vi "Generate write queue item.vi"(8 "error in (no error)":errorcluster, 11 "Abort JSON in":refnum<class "Abort JSON.lvclass">) -> (0 "error out":errorcluster, 2 "Write queue item":T1, 3 "Abort JSON out":refnum<class "Abort JSON.lvclass">)   [LabVIEW 2020, in "wamplv.lvlib" / "Abort JSON.lvclass"]
uses:
  Abort JSON.lvclass
  Abort JSON.lvclass/Abort JSON.ctl
  f2b6dabe-d674-4de4-8983-0b42131ca8da.vi
  cf9281e4-cdc7-4391-bfc3-c4a2100e25ce.vi
  TypeDefs/Transport type.ctl
  wamplv.lvlib
  WAMP Client/Private/TypeDef/Write queue item.ctl
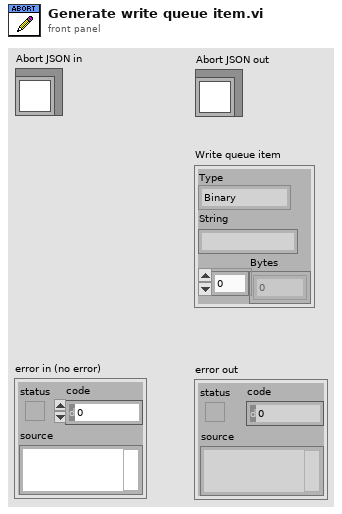
[diagram p1: front panel]
types:
  T1 = typedef "wamplv.lvlib/Write queue item.ctl" = cluster{"Type":T2, "String":string, "Bytes":u8[]}
  T2 = typedef "wamplv.lvlib/Transport type.ctl" = enum16{"Binary", "Text"}
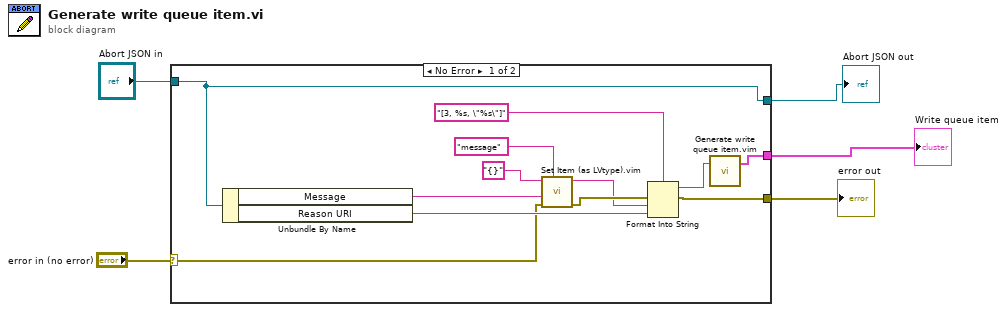
[diagram p0: block diagram]
diagram:
  n1 = case shown="No Error" "error in (no error)" {
    selector: "error in (no error)" -> [w10 w19]
    tunnel: "Abort JSON in" -> [w8 w18]
    tunnel: [w9 w19] -> w3
    tunnel: [w8 w18] -> w2
    tunnel: [w6 _] -> w1
    frame No Error {
      n2 = Unbundle By Name(w8) -> ("Message"=w12:string, "Reason URI"=w11:string)
      n3 = call "Set Item (as LVtype).vim"("$Path or Item Name"="message", "error in (no error)"=w10, "Anything"=w12, "JSON"="{}") -> ("error out"=w14:errorcluster, "<JSON>"=w13:string)  [unwired: 4 in, 1 out]
      n4 = Format Into String(format string="[3, %s, \"%s\"]", error in=w14, w13, w11) -> (resulting string=w7:string, error out=w9:errorcluster)  [unwired: 1 in]
      n5 = call "Generate write queue item.vim"("Input"=w7) -> ("Ouput"=w6:T1)  [unwired: 2 in]
    }
    frame Error {
    }
  }
  "error out" <- w3
  "Abort JSON out" <- w2
  "Write queue item" <- w1
